vi "TC test USB4718 v3.vi"() -> ()   [LabVIEW 2013]
uses:
  <vilib>/Platform/TimedLoop/XDataNode/timing_clust.ctl
  <vilib>/Platform/TimedLoop/XDataNode/nitl_modes.ctl
  <vilib>/Platform/TimedLoop/XDataNode/wakeup.ctl
  <vilib>/platform/TimedLoop/XDataNode/XDataNode.xnode
  <vilib>/Platform/TimedLoop/XDataNode/XDNodeRunTimeDep.lvlib
panel:
  out "T3 data":dbl format="%#.0f"
  out "T2 data":dbl format="%#.0f"
  in  "Stop & Open File":bool
  out "Waveform Chart":dynamicdata(graph)
  out "data file":string
  out "tdms file out":refnum<k34>
  out "CYCLES":dbl
  out "cycle":bool
  out "T3":dbl format="%#.0f"
  out "T2":dbl format="%#.0f"
  out "T1":dbl format="%#.0f"
  out "T0":dbl format="%#.0f"
  # "Note: Use ABORT button to stop program without displaying data file."
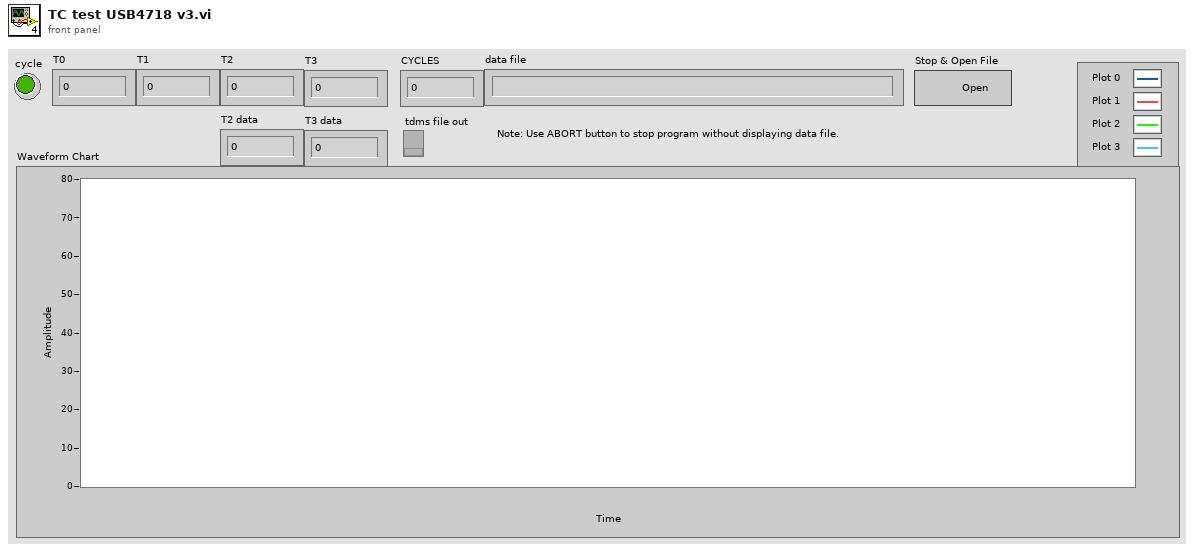
[diagram p1: front panel]
types:
  T1 = enum16{"open", "open or create", "create or replace", "create", "open (read-only)"}
  T2 = typedef "XDNodeRunTimeDep.lvlib/timing_clust.ctl" = cluster{"Expected End [f-1]":u64, "Actual End [f-1]":u64, "Finished Late? [f-1]":bool, "Expected End [i-1]":u64, "Actual End [i-1]":u64, "Finished Late? [i-1]":bool, "Expected Start [i]":u64, "Actual Start [i]":u64, "Expected Start [f]":u64, "Actual Start [f]":u64, "Source Name":string, "Structure Name":string, "Period":i64, "Deadline":i64, "Offset":i64, "Start":i64, "Priority":i32, "Timeout":i32, "Mode":T3, "Wakeup Reason":T4, "Error":errorcluster, "Source Type":string, "Secondary Source Type":string, "Global End Time":u64, "Global Start Time":u64, "Frame Duration":u64, "Iteration Duration":u64, "Assigned CPU":i32, "I/O Scan Engine Mode":u32}
  T3 = typedef "XDNodeRunTimeDep.lvlib/nitl_modes.ctl" = enum32{"No Change", "Process missed periods, maintain original phase", "Discard missed periods, maintain original phase", "Process missed periods, ignore original phase", "Discard missed periods, ignore original phase"}
  T4 = typedef "XDNodeRunTimeDep.lvlib/wakeup.ctl" = enum32{"Normal", "Aborted", "Asynchronous wakeup", "Timing source error", "Timed loop error", "Timeout"}
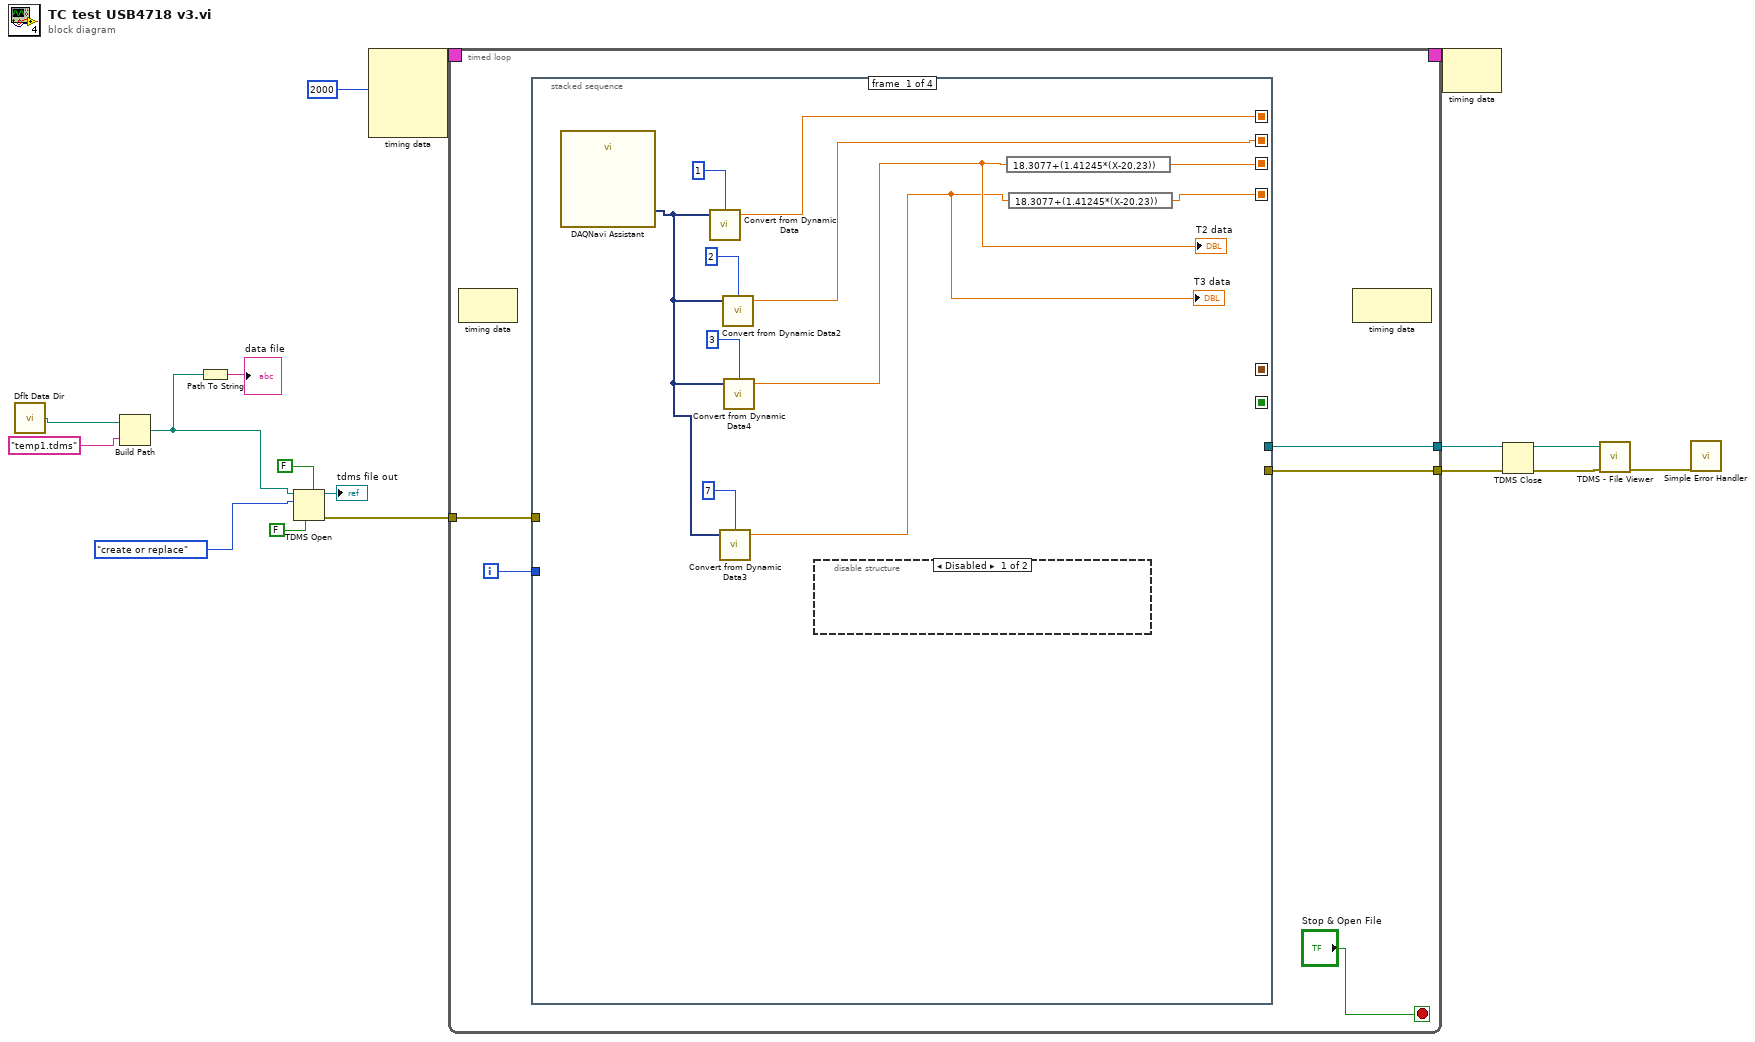
[diagram p0: block diagram]
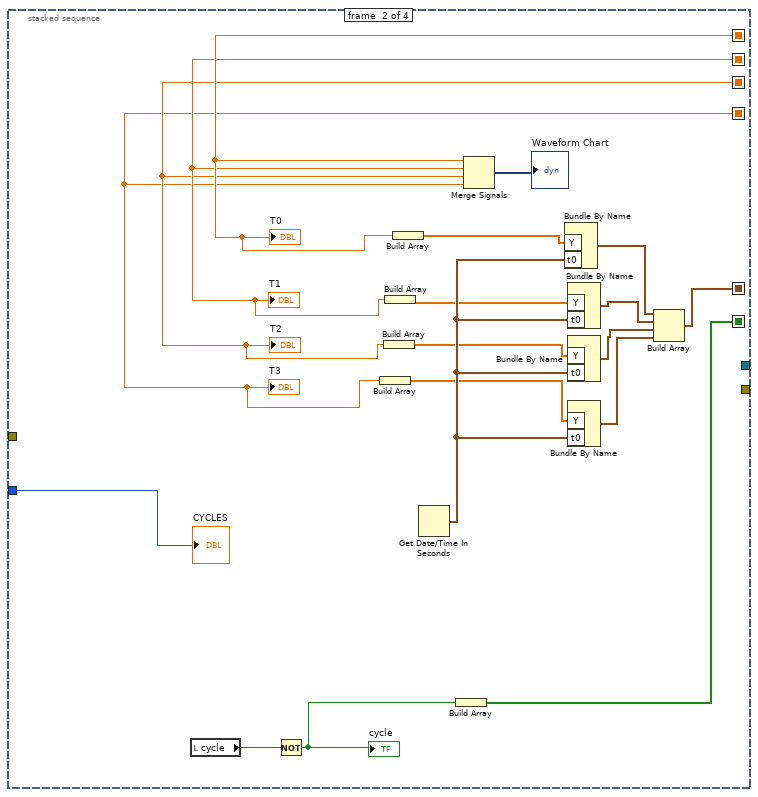
[diagram p3: hidden frame]
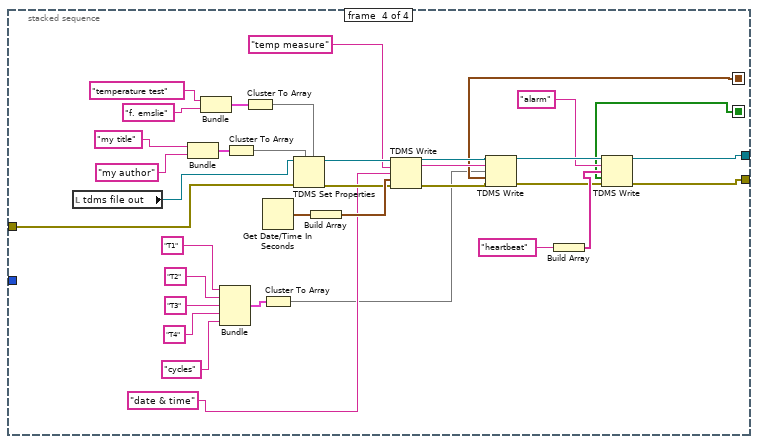
[diagram p5: hidden frame]
diagram:
  n1 = call <vilib>:"Dflt Data Dir.vi"() -> ("App:Default Data Directory"=w5:path)
  n2 = Build Path(base path=w5, name or relative path="temp1.tdms") -> (appended path=w6:path)
  n3 = Path To String(path=w6) -> (string=→"data file":string)
  n4 = TDMS Open(5:FALSE ("create index file? (T)"), 6:FALSE ("disable buffering? (T)"), 10:T1."create or replace" ("operation (0:open)"), 11:w6) -> (0:w13:errorcluster, 3:→"tdms file out":refnum<k34>)  [unwired: 3 in]
  n5 = node-c288(2000) -> (w17:T2)  [unwired: 3 in]
  n6 = timed-loop {
    timing: w17 -> [_]
    timing-out: [_] -> w16
    tunnel: w13 -> [w21]
    tunnel: [w20] -> w12
    tunnel: [w19] -> w11
    i -> [w22]
    stop <- "Stop & Open File" stop-if-true
    n7 = node-c288() -> ()  [unwired: 1 in, 1 out]
    n8 = stacked-sequence {
      seq-local: [_ w47 _ _] -> [_ _ _ w63]
      seq-local: [_ w43 _ _] -> [_ _ _ w58]
      seq-local: [w28 _ _ _] -> [_ w37 _ _]
      seq-local: [w27 _ _ _] -> [_ w36 _ _]
      seq-local: [w26 _ _ _] -> [_ w35 _ _]
      seq-local: [w25 _ _ _] -> [_ w34 _ _]
      tunnel: w22 -> [_ w51 _ _]
      tunnel: w21 -> [_ _ _ w72]
      tunnel: [_ _ _ w56] -> w20
      tunnel: [_ _ _ w55] -> w19
      frame #0 {
        n9 = call "DAQNavi Assistant"() -> ("data out(DDT)"=w29:dynamicdata)  [unwired: 26 in, 1 out]
        n10 = call "Convert from Dynamic Data"("Dynamic Data Type"=w29, "Channel"=1) -> ("Scalar"=w28:dbl)  [unwired: 2 in]
        n11 = call "Convert from Dynamic Data3"("Dynamic Data Type"=w29, "Channel"=7) -> ("Scalar"=w23:dbl)  [unwired: 2 in]
        "T3 data" <- w23
        n12 = call "Convert from Dynamic Data2"("Dynamic Data Type"=w29, "Channel"=2) -> ("Scalar"=w27:dbl)  [unwired: 2 in]
        n13 = call "Convert from Dynamic Data4"("Dynamic Data Type"=w29, "Channel"=3) -> ("Scalar"=w24:dbl)  [unwired: 2 in]
        "T2 data" <- w24
        n14 = disable-structure shown="Disabled" {
          frame Disabled {
          }
          frame Enabled {
          }
        }
        n15 = expression code="18.3077+(1.41245*(X-20.23))"(w24) -> (w26:dbl)
        n16 = expression code="18.3077+(1.41245*(X-20.23))"(w23) -> (w25:dbl)
      }
      frame #1 {
        n17 = local read "cycle"() -> (w52:bool)
        n18 = Not(x=w52) -> (.not. x?=w50:bool)
        "cycle" <- w50
        n19 = Build Array(w34) -> (w38:dbl[])
        n20 = Build Array(w35) -> (w39:dbl[])
        n21 = Build Array(w36) -> (w40:dbl[])
        n22 = Build Array(w37) -> (w41:dbl[])
        n23 = Get Date/Time In Seconds() -> (seconds since 1Jan1904=w48:timestamp)
        n24 = Build Array(w50) -> (w43:bool[])
        n25 = Merge Signals(w37, w36, w35, w34) -> (→"Waveform Chart":dynamicdata)
        n26 = Bundle By Name("Y"=w41, "t0"=w48) -> (w49:waveform(dbl))  [unwired: 1 in]
        n27 = Bundle By Name("Y"=w40, "t0"=w48) -> (w46:waveform(dbl))  [unwired: 1 in]
        n28 = Bundle By Name("Y"=w39, "t0"=w48) -> (w45:waveform(dbl))  [unwired: 1 in]
        n29 = Bundle By Name("Y"=w38, "t0"=w48) -> (w44:waveform(dbl))  [unwired: 1 in]
        n30 = Build Array(w49, w46, w45, w44) -> (w47:waveform(dbl)[])
        "T1" <- w36
        "T3" <- w34
        "T0" <- w37
        "T2" <- w35
        "CYCLES" <- w51
      }
      frame #2 {
      }
      frame #3 {
        n31 = local read "tdms file out"() -> (w54:refnum<k34>)
        n32 = Bundle("my title", "my author") -> (w75:cluster{string, string})  [unwired: 1 in]
        n33 = Bundle("temperature test", "f. emslie") -> (w78:cluster{string, string})  [unwired: 1 in]
        n34 = Bundle("T1", "T2", "T3", "T4", "cycles") -> (w83:cluster{string, string, string, string, string})  [unwired: 1 in]
        n35 = Cluster To Array(cluster=w75) -> (array=w76:string[])
        n36 = Cluster To Array(cluster=w78) -> (array=w74:string[])
        n37 = Get Date/Time In Seconds() -> (seconds since 1Jan1904=w81:timestamp)
        n38 = Cluster To Array(cluster=w83) -> (array=w53:string[])
        n39 = TDMS Set Properties(5:w74, 7:w76, 8:w72, 11:w54) -> (0:w70:errorcluster, 3:w69:refnum<k34>)  [unwired: 2 in, 2 out]
        n40 = Build Array(w81) -> (w71:timestamp[])
        n41 = TDMS Write(0:w69, 5:"temp measure", 7:"date & time", 9:w71, 11:w70) -> (4:w65:refnum<k34>, 6:w64:string, 15:w66:errorcluster)  [unwired: 1 in, 1 out]
        n42 = TDMS Write(0:w65, 5:w64, 7:w53, 9:w63, 11:w66) -> (4:w62:refnum<k34>, 15:w57:errorcluster)  [unwired: 1 in, 2 out]
        n43 = Build Array("heartbeat") -> (w59:string[])
        n44 = TDMS Write(0:w62, 5:"alarm", 7:w59, 9:w58, 11:w57) -> (4:w56:refnum<k34>, 15:w55:errorcluster)  [unwired: 1 in, 2 out]
      }
    }
    n45 = node-c288() -> ()  [unwired: 1 in, 1 out]
  }
  n46 = node-c288(w16) -> ()  [unwired: 1 out]
  n47 = TDMS Close(8:w11, 11:w12) -> (0:w4:errorcluster, 3:w2:path)
  n48 = call <vilib>:"TDMS - File Viewer.vi"("error in (no error)"=w4, "file path"=w2) -> ("error out"=w3:errorcluster)  [unwired: 4 in, 1 out]
  n49 = call <vilib>:"Simple Error Handler.vi"("error in (no error)"=w3) -> ()  [unwired: 4 in, 5 out]
